vi "test.vi"() -> ()   [LabVIEW 2012]
panel:
  out "String 4":string
  out "Numeric":dbl
  out "receive buffer":string
  out "error out":errorcluster
  in  "Radio Buttons":T1(radio)
  out "String 3":string
  out "String 2":string
  out "String":string
  in  "VISA resource name":refnum<visa-resource-name>
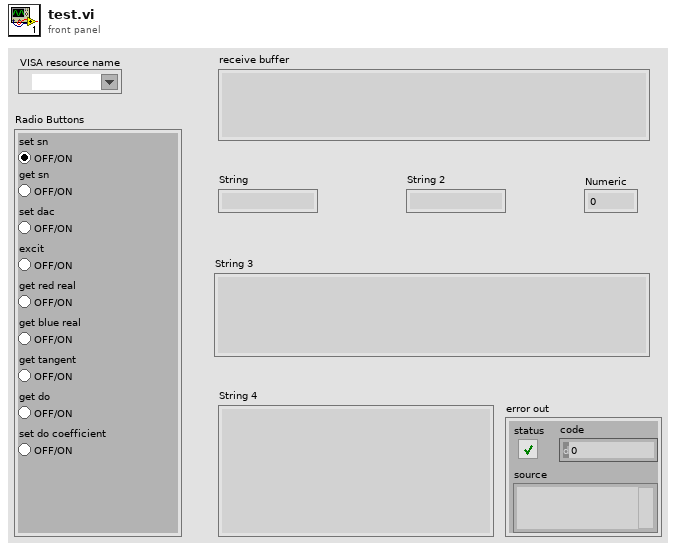
[diagram p1: front panel]
types:
  T1 = enum32{"set sn", "get sn", "set dac", "excit", "get red real", "get blue real", "get tangent", "get do", "set do coefficient"}
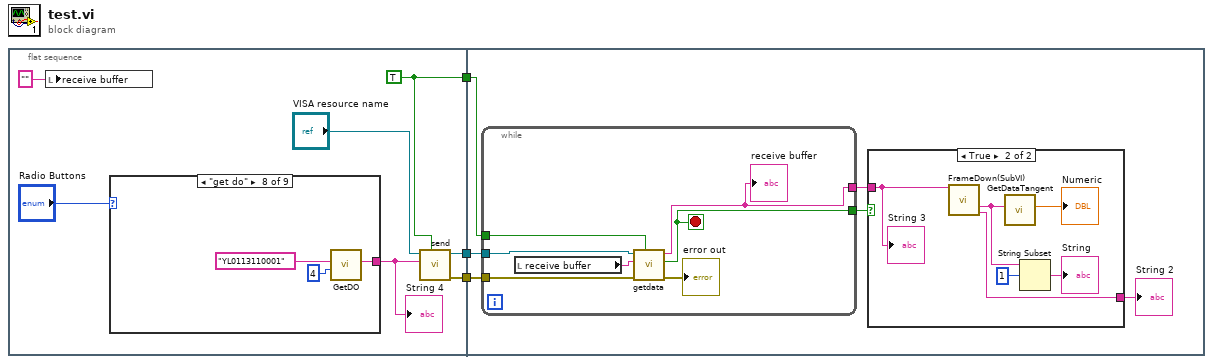
[diagram p0: block diagram]
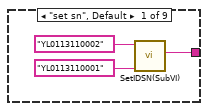
[diagram p2: hidden frame]
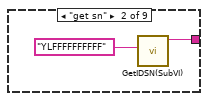
[diagram p3: hidden frame]
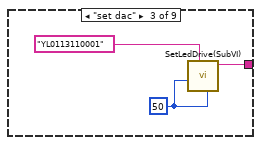
[diagram p4: hidden frame]
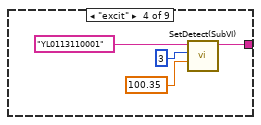
[diagram p5: hidden frame]
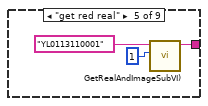
[diagram p6: hidden frame]
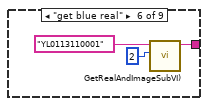
[diagram p7: hidden frame]
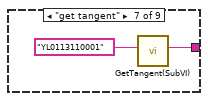
[diagram p8: hidden frame]
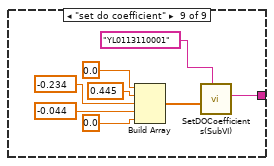
[diagram p9: hidden frame]
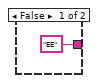
[diagram p10: hidden frame]
diagram:
  n1 = flat-sequence {
    tunnel: [w10] -> w3
    tunnel: [w8] -> w2
    tunnel: [w7] -> w1
    tunnel: w3 -> [w47]
    tunnel: w2 -> [w46]
    tunnel: w1 -> [w45]
    frame #0 {
      w10 = TRUE
      n2 = local write "receive buffer"("") -> ()
      n3 = case shown="\"get do\"" "Radio Buttons" {
        tunnel: [w11 w14 w18 w22 w23 w26 w30 w32 w41] -> w4
        frame "set sn", Default {
          n4 = call "SetIDSN(SubVI).vi"("input sn"="YL0113110001", "sn"="YL0113110002") -> ("output frame"=w11:string)  [unwired: 9 in]
        }
        frame "get sn" {
          n5 = call "GetIDSN(SubVI).vi"("sn"="YLFFFFFFFFFF") -> ("output frame"=w14:string)  [unwired: 10 in]
        }
        frame "set dac" {
          w16 = 50
          n6 = call "SetLedDrive(SubVI).vi"("blue dac"=w16, "sn"="YL0113110001", "red dac"=w16) -> ("String"=w18:string)  [unwired: 8 in]
        }
        frame "excit" {
          n7 = call "SetDetect(SubVI).vi"("pressure"=100.35, "led selected"=3, "sn"="YL0113110001") -> ("output frame"=w22:string)  [unwired: 8 in]
        }
        frame "get red real" {
          n8 = call "GetRealAndImageSubVI).vi"("byte data"=1, "sn"="YL0113110001") -> ("output frame"=w23:string)  [unwired: 9 in]
        }
        frame "get blue real" {
          n9 = call "GetRealAndImageSubVI).vi"("byte data"=2, "sn"="YL0113110001") -> ("output frame"=w26:string)  [unwired: 9 in]
        }
        frame "get tangent" {
          n10 = call "GetTangent(SubVI).vi"("sn"="YL0113110001") -> ("output frame"=w30:string)  [unwired: 10 in]
        }
        frame "get do" {
          n11 = call "GetDO.vi"("select"=4, "sn"="YL0113110001") -> ("output frame"=w32:string)  [unwired: 9 in]
        }
        frame "set do coefficient" {
          n12 = Build Array(0.0, 0.445, -0.234, -0.044, 0.0) -> (w39:dbl[])
          n13 = call "SetDOCoefficients(SubVI).vi"("sn"="YL0113110001", "L"=w39) -> ("output frame"=w41:string)  [unwired: 9 in]
        }
      }
      "String 4" <- w4
      n14 = call "send.vi"("condition"=w10, "input"=w4, "port"="VISA resource name") -> ("error out"=w8:errorcluster, "VISA resource name"=w7:refnum<visa-resource-name>)  [unwired: 6 in, 1 out]
    }
    frame #1 {
      n15 = while {
        tunnel: w47 -> [w54]
        tunnel: w46 -> [w52]
        tunnel: w45 -> [w51]
        tunnel: [w50] -> w44
        tunnel: [w49] -> w42
        stop <- w50 stop-if-true
        n16 = local read "receive buffer"() -> (w48:string)
        n17 = call "getdata.vi"("condition"=w54, "error in (no error)"=w52, "inputdata"=w48, "port"=w51) -> ("error out"=→"error out":errorcluster, "end"=w50:bool, "outputdata"=w49:string)  [unwired: 4 in, 1 out]
        "receive buffer" <- w49
      }
      n18 = case shown="True" w44 {
        tunnel: w42 -> [_ w60]
        tunnel: ["EE" w58] -> w43
        frame False {
        }
        frame True {
          n19 = call "FrameDown(SubVI).vi"("input frame"=w60) -> ("data"=w57:string, "result"=w58:string)  [unwired: 4 in, 9 out]
          n20 = call "GetDataTangent.vi"("input data"=w57) -> ("tangent"=→"Numeric":dbl)  [unwired: 10 in]
          n21 = String Subset(string=w57, offset (0)=1) -> (substring=→"String":string)  [unwired: 1 in]
          "String 3" <- w60
        }
      }
      "String 2" <- w43
    }
  }
